vi "Catapult Control Single Solenoid.vi"(6 "Sensor Analog Status":sgl=5.0 format="%#_13g", 7 "Sensor Digital Status":bool, 8 "Error In":errorcluster, 9 "Second Action":T1=enum."Hold", 10 "First Action":T1=enum."Hold", 11 "CatapultDevRefIn":T2={"Catapult State Reference"=refnum, "SolenoidDevRef"={"DevStatus"={"status"=FALSE, "code"=0, "source"=""}, "Pneumatics Control Module"=208, "Forward Solenoid Channel"=enum."Invalid", "Reverse Solenoid Channel"=enum."Invalid"}, "Catapult Configuration Reference"=refnum}) -> (1 "Action Complete":bool=TRUE, 2 "Solenoid Position":bool, 3 "CatapultDevRefOut":T2={"Catapult State Reference"=refnum, "SolenoidDevRef"={"DevStatus"={"status"=FALSE, "code"=0, "source"=""}, "Pneumatics Control Module"=208, "Forward Solenoid Channel"=enum."Invalid", "Reverse Solenoid Channel"=enum."Invalid"}, "Catapult Configuration Reference"=refnum})   [LabVIEW 2015]
uses:
  <userlib>/836 Library/Pneumatics/Catapult/836_CatapultActions.ctl
  <userlib>/836 Library/Pneumatics/Catapult/836_CatapultDevRef.ctl
  <userlib>/836 Library/Pneumatics/Catapult/Catapult State.ctl
  <userlib>/836 Library/Pneumatics/Catapult/CatapultStateMachine.ctl
  <vilib>/Rock Robotics/WPI/Solenoid/WPI_SolenoidDevRef.ctl
  <vilib>/Rock Robotics/WPI/Solenoid/WPI_SolenoidChannel.ctl
  <userlib>/836 Library/Pneumatics/Catapult/Catapult Configuration.ctl
  <vilib>/Rock Robotics/WPI/Solenoid/WPI_SolenoidValue.ctl
  <vilib>/Rock Robotics/WPI/Solenoid/WPI_SolenoidSetEnum.vi
panel:
  out "Error Out":errorcluster
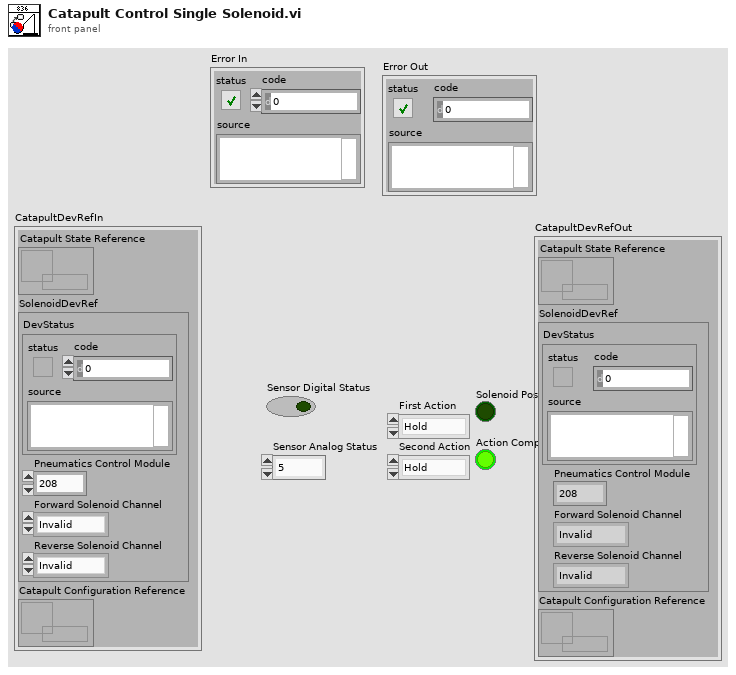
[diagram p1: front panel]
types:
  T1 = typedef "836_CatapultActions.ctl" = enum8{"Fire", "Fire Timed", "Fire Analog", "Fire Digital", "Retract", "Retract Timed", "Retract Analog", "Retract Digital", "Hold", "Toggle", "Toggle Timed", "Toggle Analog", "Toggle Digital"}
  T2 = typedef "836_CatapultDevRef.ctl" = cluster{"Catapult State Reference":refnum<data-value>, "SolenoidDevRef":T3, "Catapult Configuration Reference":refnum<data-value>}
  T3 = typedef "WPI_SolenoidDevRef.ctl" = cluster{"DevStatus":errorcluster, "Pneumatics Control Module":u8, "Forward Solenoid Channel":T4, "Reverse Solenoid Channel":T4}
  T4 = typedef "WPI_SolenoidChannel.ctl" = enum8{"Solenoid 0", "Solenoid 1", "Solenoid 2", "Solenoid 3", "Solenoid 4", "Solenoid 5", "Solenoid 6", "Solenoid 7", "Invalid"}
  T5 = typedef "WPI_SolenoidValue.ctl" = enum16{"Off", "On", "Forward", "Reverse"}
  T6 = typedef "CatapultStateMachine.ctl" = enum8{"Status", "Forward", "Back", "Timed Forward", "Timed Back", "Analog Forwad", "Analog Back", "Digital Forward", "Digital Back", "Off"}
  T7 = typedef "Catapult State.ctl" = cluster{"Position":bool, "Initialize":bool, "First Action?":bool, "Current State":T6, "Multiuse Timer":u32, "Second Action":T1}
  T8 = typedef "Catapult Configuration.ctl" = cluster{"Time Forward":u32, "Time Back":u32, "Digital Forward Samples":u32, "Digital Backward Samples":u32, "Analog Forward Settling Time":u32, "Analog Backward Settling Time":u32, "Analog Forward Threshold":sgl, "Analog Backward Threshold":sgl}
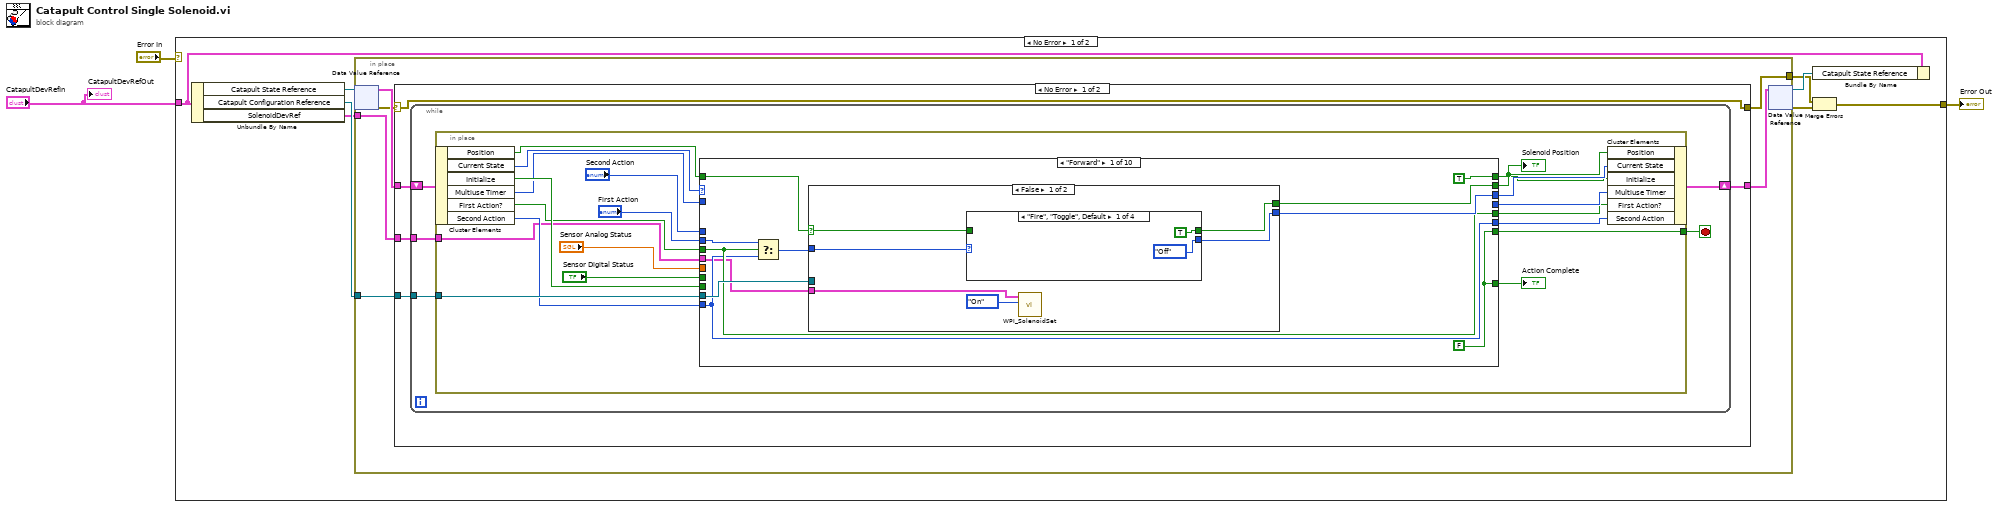
[diagram p0: block diagram]
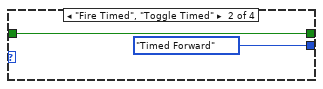
[diagram p2: hidden frame]
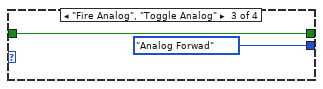
[diagram p3: hidden frame]
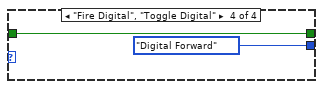
[diagram p4: hidden frame]
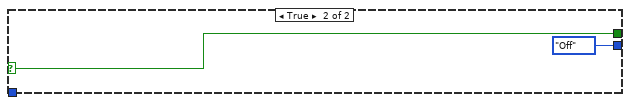
[diagram p5: hidden frame]
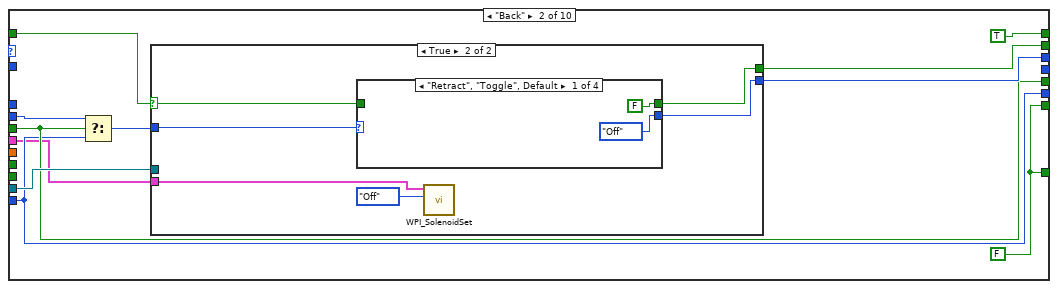
[diagram p6: hidden frame]
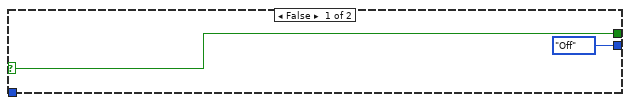
[diagram p7: hidden frame]
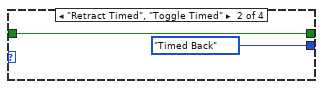
[diagram p8: hidden frame]
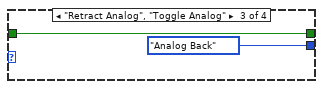
[diagram p9: hidden frame]
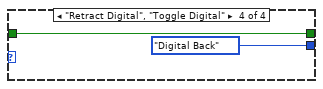
[diagram p10: hidden frame]
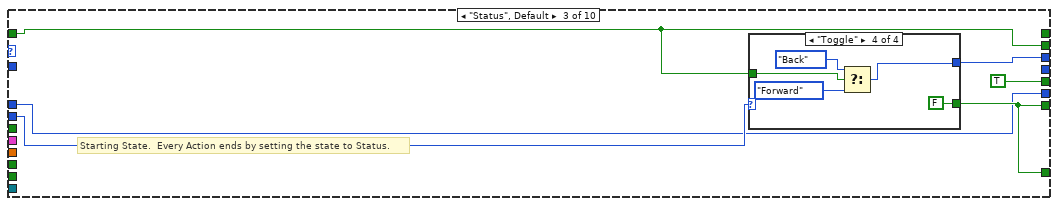
[diagram p11: hidden frame]
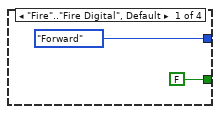
[diagram p12: hidden frame]
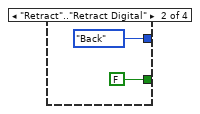
[diagram p13: hidden frame]
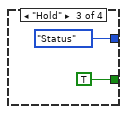
[diagram p14: hidden frame]
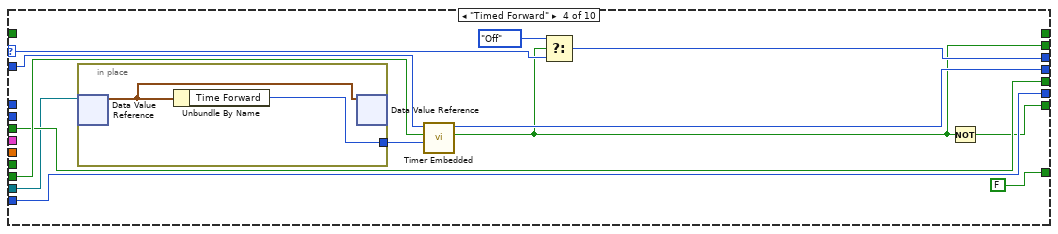
[diagram p15: hidden frame]
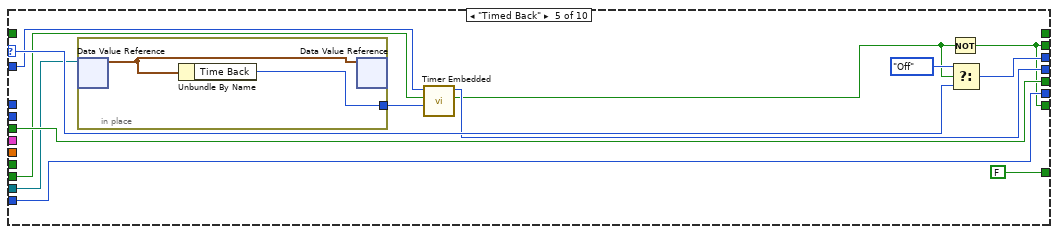
[diagram p16: hidden frame]
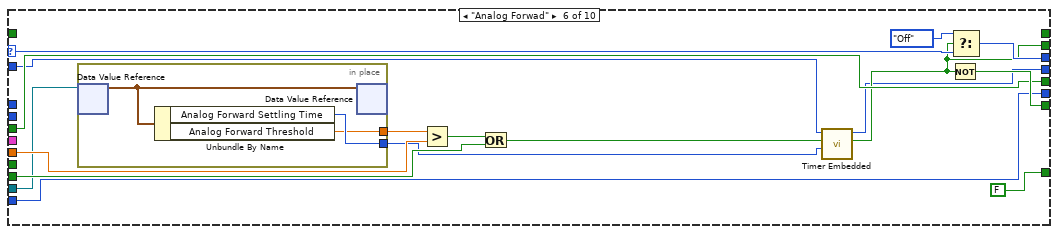
[diagram p17: hidden frame]
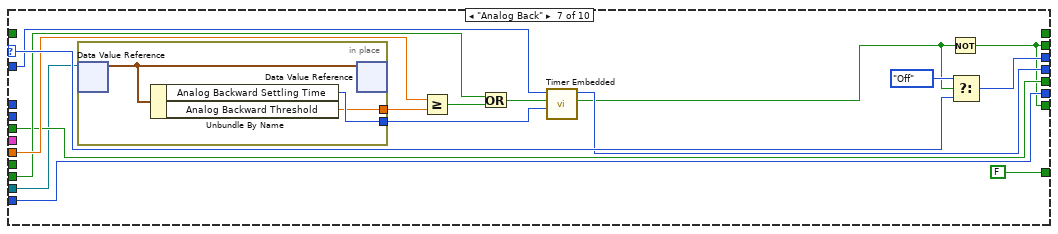
[diagram p18: hidden frame]
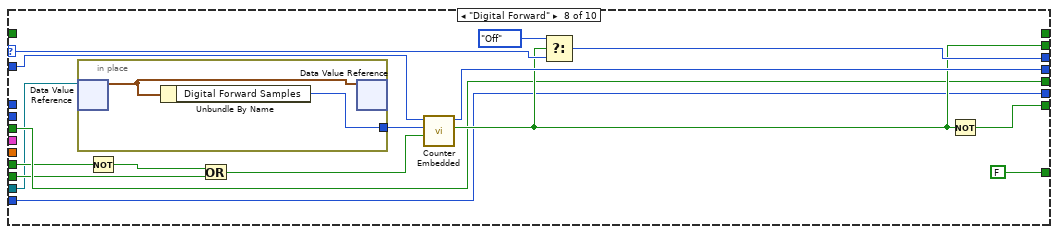
[diagram p19: hidden frame]
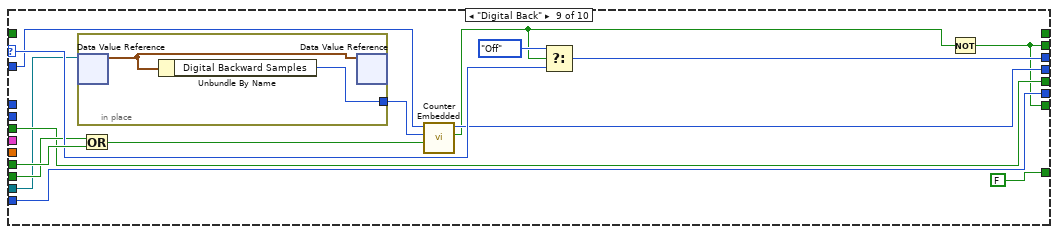
[diagram p20: hidden frame]
diagram:
  n1 = case shown="No Error" "Error In" {
    selector: "Error In" -> [_ w241]
    tunnel: "CatapultDevRefIn" -> [w8 _]
    tunnel: [w5 w241] -> w2
    frame No Error {
      n2 = Unbundle By Name(w8) -> ("Catapult State Reference"=w11:refnum<data-value>, "Catapult Configuration Reference"=w10:refnum<data-value>, "SolenoidDevRef"=w4:T3)
      n3 = in-place {
        in-place-border: w10 -> [w16]
        in-place-border: [w13] -> w7
        in-place-border: w4 -> [w12]
        n4 = in-place-dvr #1(w11) -> (w17:T7, w14:errorcluster)
        n5 = case shown="No Error" w14 {
          selector: w14 -> [w20 w239]
          tunnel: w17 -> [w22 w240]
          tunnel: w16 -> [w21 _]
          tunnel: [w19 w240] -> w15
          tunnel: [w20 w239] -> w13
          tunnel: w12 -> [w18 _]
          frame No Error {
            n6 = while {
              tunnel: w21 -> [w26]
              shift-right: [w24] -> w19
              shift-left: w22 -> [w27]
              tunnel: w18 -> [w23]
              stop <- w25 stop-if-true
              n7 = in-place {
                in-place-border: w26 -> [w40]
                in-place-border: [w36] -> w25
                in-place-border: w23 -> [w28]
                n8 = in-place-cluster #2(w27) -> ("Position"=w44:bool, "Current State"=w38:T6, "Initialize"=w43:bool, "Multiuse Timer"=w39:u32, "First Action?"=w31:bool, "Second Action"=w34:T1)
                n9 = case shown="\"Forward\"" w38 {
                  selector: w38 -> [_ _ _ w130 w145 w162 w184 w202 w218 _]
                  tunnel: [w49 w76 w105 w122 w136 w159 w172 w197 w209 w230] -> w36
                  tunnel: w44 -> [w56 w84 w102 _ _ _ _ _ _ w232]
                  tunnel: [w58 w85 w102 w121 w136 w153 w172 w198 w209 w232] -> w42
                  tunnel: "Sensor Digital Status" -> [_ _ _ _ _ _ _ w193 w220 _]
                  tunnel: [w57 w83 w106 w131 w146 w165 w185 w204 w221 w231] -> w41
                  tunnel: "Sensor Analog Status" -> [_ _ _ _ _ w164 w183 _ _ _]
                  tunnel: w43 -> [_ _ _ w126 w140 w160 w180 w191 w217 _]
                  tunnel: [w49 w76 w105 FALSE FALSE FALSE FALSE FALSE FALSE w230] -> w45
                  tunnel: w39 -> [_ _ _ w127 w139 w155 w175 w199 w213 _]
                  tunnel: [_ _ _ w128 w138 w152 w174 w200 w211 _] -> w35
                  tunnel: w40 -> [w55 w82 _ w120 w135 w151 w171 w190 w208 _]
                  tunnel: [TRUE TRUE _ _ _ _ _ _ _ TRUE] -> w37
                  tunnel: "First Action" -> [w53 w80 w107 _ _ _ _ _ _ _]
                  tunnel: w34 -> [w50 w77 _ w123 w141 w156 w177 w194 w214 w226]
                  tunnel: [w51 w78 TRUE w124 w142 w157 w178 w195 w215 FALSE ("First Action?")] -> w32
                  tunnel: w31 -> [w51 w78 _ w124 w142 w157 w178 w195 w215 w224]
                  tunnel: "Second Action" -> [_ _ w103 _ _ _ _ _ _ _]
                  tunnel: [w50 w77 w103 w123 w141 w156 w177 w194 w214 w226] -> w29
                  tunnel: w28 -> [w48 w75 _ _ _ _ _ _ _ _]
                  frame "Forward" {
                    w49 = FALSE
                    n10 = Select(t=w53, s=w51, f=w50) -> (s? t:f=w52:T1)
                    n11 = case shown="False" w56 {
                      selector: w56 -> [w62 w74]
                      tunnel: [w64 w74] -> w58
                      tunnel: [w63 CatapultStateMachine."Off" ("f")] -> w57
                      tunnel: w55 -> [_ _]
                      tunnel: w52 -> [w60 _]
                      tunnel: w48 -> [w59 _]
                      frame False {
                        n12 = case shown="\"Fire\", \"Toggle\", Default" w60 {
                          tunnel: [CatapultStateMachine."Off" ("Current State") CatapultStateMachine."Timed Forward" ("Current State") CatapultStateMachine."Analog Forwad" ("Current State") CatapultStateMachine."Digital Forward" ("Current State")] -> w63
                          tunnel: w62 -> [_ w68 w70 w72]
                          tunnel: [TRUE w68 w70 w72] -> w64
                          frame "Fire", "Toggle", Default {
                          }
                          frame "Fire Timed", "Toggle Timed" {
                          }
                          frame "Fire Analog", "Toggle Analog" {
                          }
                          frame "Fire Digital", "Toggle Digital" {
                          }
                        }
                        n13 = call-poly <vilib>:"WPI_SolenoidSet.vi"("Value"=WPI_SolenoidValue."On" ("Value 3"), "SolenoidDevRef"=w59) -> ()  [unwired: 8 in, 2 out]
                      }
                      frame True {
                      }
                    }
                  }
                  frame "Back" {
                    w76 = FALSE
                    n14 = Select(t=w80, s=w78, f=w77) -> (s? t:f=w79:T1)
                    n15 = case shown="True" w84 {
                      selector: w84 -> [w87 w91]
                      tunnel: [w87 w93] -> w85
                      tunnel: [CatapultStateMachine."Off" ("f") w92] -> w83
                      tunnel: w82 -> [_ _]
                      tunnel: w79 -> [_ w89]
                      tunnel: w75 -> [_ w88]
                      frame False {
                      }
                      frame True {
                        n16 = case shown="\"Retract\", \"Toggle\", Default" w89 {
                          tunnel: [CatapultStateMachine."Off" ("Current State") CatapultStateMachine."Timed Back" ("Current State") CatapultStateMachine."Analog Back" ("Current State") CatapultStateMachine."Digital Back" ("Current State")] -> w92
                          tunnel: [FALSE w97 w99 w101] -> w93
                          tunnel: w91 -> [_ w97 w99 w101]
                          frame "Retract", "Toggle", Default {
                          }
                          frame "Retract Timed", "Toggle Timed" {
                          }
                          frame "Retract Analog", "Toggle Analog" {
                          }
                          frame "Retract Digital", "Toggle Digital" {
                          }
                        }
                        n17 = call-poly <vilib>:"WPI_SolenoidSet.vi"("Value"=WPI_SolenoidValue."Off" ("Value 3"), "SolenoidDevRef"=w88) -> ()  [unwired: 8 in, 2 out]
                      }
                    }
                  }
                  frame "Status", Default {
                    # "Starting State.  Every Action ends by setting the state to Status."
                    n18 = case shown="\"Toggle\"" w107 {
                      tunnel: [CatapultStateMachine."Forward" ("Current State") CatapultStateMachine."Back" ("Current State") CatapultStateMachine."Status" ("Current State") w114] -> w106
                      tunnel: [FALSE FALSE TRUE FALSE] -> w105
                      tunnel: w102 -> [_ _ _ w117]
                      frame "Fire".."Fire Digital", Default {
                      }
                      frame "Retract".."Retract Digital" {
                      }
                      frame "Hold" {
                      }
                      frame "Toggle" {
                        n19 = Select(t=CatapultStateMachine."Back" ("Current State"), s=w117, f=CatapultStateMachine."Forward" ("Current State")) -> (s? t:f=w114:T6)
                      }
                    }
                  }
                  frame "Timed Forward" {
                    n20 = in-place {
                      in-place-border: [w133] -> w119
                      n21 = in-place-dvr #3(w120) -> (w132:T8)  [unwired: 1 out]
                      n22 = Unbundle By Name(w132) -> ("Time Forward"=w133:u32)
                      n23 = in-place-dvr #3(w132) -> ()  [unwired: 2 out]
                    }
                    n24 = call <userlib>:"Timer Embedded.vi"("Time Limit"=w119, "Reset"=w126, "Start Time In"=w127) -> ("Time Limit Passed"=w121:bool, "Start Time Out"=w128:u32)  [unwired: 7 in]
                    n25 = Select(t=CatapultStateMachine."Off" ("Current State"), s=w121, f=w130) -> (s? t:f=w131:T6)
                    n26 = Not(x=w121) -> (.not. x?=w122:bool)
                  }
                  frame "Timed Back" {
                    n27 = in-place {
                      in-place-border: [w148] -> w134
                      n28 = in-place-dvr #4(w135) -> (w147:T8)  [unwired: 1 out]
                      n29 = Unbundle By Name(w147) -> ("Time Back"=w148:u32)
                      n30 = in-place-dvr #4(w147) -> ()  [unwired: 2 out]
                    }
                    n31 = call <userlib>:"Timer Embedded.vi"("Time Limit"=w134, "Reset"=w140, "Start Time In"=w139) -> ("Time Limit Passed"=w137:bool, "Start Time Out"=w138:u32)  [unwired: 7 in]
                    n32 = Not(x=w137) -> (.not. x?=w136:bool)
                    n33 = Select(t=CatapultStateMachine."Off" ("Current State"), s=w137, f=w145) -> (s? t:f=w146:T6)
                  }
                  frame "Analog Forwad" {
                    n34 = in-place {
                      in-place-border: [w168] -> w150
                      in-place-border: [w167] -> w149
                      n35 = in-place-dvr #5(w151) -> (w166:T8)  [unwired: 1 out]
                      n36 = Unbundle By Name(w166) -> ("Analog Forward Settling Time"=w168:u32, "Analog Forward Threshold"=w167:sgl)
                      n37 = in-place-dvr #5(w166) -> ()  [unwired: 2 out]
                    }
                    n38 = Greater?(x=w149, y=w164) -> (0:w163:bool)
                    n39 = Or(x=w163, y=w160) -> (x .or. y?=w154:bool)
                    n40 = call <userlib>:"Timer Embedded.vi"("Time Limit"=w150, "Reset"=w154, "Start Time In"=w155) -> ("Time Limit Passed"=w153:bool, "Start Time Out"=w152:u32)  [unwired: 7 in]
                    n41 = Not(x=w153) -> (.not. x?=w159:bool)
                    n42 = Select(t=CatapultStateMachine."Off" ("Current State"), s=w153, f=w162) -> (s? t:f=w165:T6)
                  }
                  frame "Analog Back" {
                    n43 = in-place {
                      in-place-border: [w188] -> w169
                      in-place-border: [w187] -> w170
                      n44 = in-place-dvr #6(w171) -> (w186:T8)  [unwired: 1 out]
                      n45 = Unbundle By Name(w186) -> ("Analog Backward Settling Time"=w188:u32, "Analog Backward Threshold"=w187:sgl)
                      n46 = in-place-dvr #6(w186) -> ()  [unwired: 2 out]
                    }
                    n47 = Greater Or Equal?(x=w183, y=w170) -> (x >= y?=w182:bool)
                    n48 = Or(x=w180, y=w182) -> (x .or. y?=w176:bool)
                    n49 = call <userlib>:"Timer Embedded.vi"("Time Limit"=w169, "Reset"=w176, "Start Time In"=w175) -> ("Time Limit Passed"=w173:bool, "Start Time Out"=w174:u32)  [unwired: 7 in]
                    n50 = Not(x=w173) -> (.not. x?=w172:bool)
                    n51 = Select(t=CatapultStateMachine."Off" ("Current State"), s=w173, f=w184) -> (s? t:f=w185:T6)
                  }
                  frame "Digital Forward" {
                    n52 = in-place {
                      in-place-border: [w206] -> w189
                      n53 = in-place-dvr #7(w190) -> (w205:T8)  [unwired: 1 out]
                      n54 = Unbundle By Name(w205) -> ("Digital Forward Samples"=w206:u32)
                      n55 = in-place-dvr #7(w205) -> ()  [unwired: 2 out]
                    }
                    n56 = Not(x=w193) -> (.not. x?=w192:bool)
                    n57 = Or(x=w192, y=w191) -> (x .or. y?=w203:bool)
                    n58 = call <userlib>:"Counter Embedded.vi"("Reset"=w203, "Digital Limit"=w189, "Digital Count In"=w199) -> ("Limit Reached"=w198:bool, "Digital Count Out"=w200:u32)  [unwired: 7 in]
                    n59 = Select(t=CatapultStateMachine."Off" ("Current State"), s=w198, f=w202) -> (s? t:f=w204:T6)
                    n60 = Not(x=w198) -> (.not. x?=w197:bool)
                  }
                  frame "Digital Back" {
                    n61 = in-place {
                      in-place-border: [w223] -> w207
                      n62 = in-place-dvr #8(w208) -> (w222:T8)  [unwired: 1 out]
                      n63 = Unbundle By Name(w222) -> ("Digital Backward Samples"=w223:u32)
                      n64 = in-place-dvr #8(w222) -> ()  [unwired: 2 out]
                    }
                    n65 = Or(x=w217, y=w220) -> (x .or. y?=w212:bool)
                    n66 = call <userlib>:"Counter Embedded.vi"("Reset"=w212, "Digital Limit"=w207, "Digital Count In"=w213) -> ("Limit Reached"=w210:bool, "Digital Count Out"=w211:u32)  [unwired: 7 in]
                    n67 = Select(t=CatapultStateMachine."Off" ("Current State"), s=w210, f=w218) -> (s? t:f=w221:T6)
                    n68 = Not(x=w210) -> (.not. x?=w209:bool)
                  }
                  frame "Off" {
                    n69 = Select(t=w226, s=w224, f=836_CatapultActions."Hold") -> (s? t:f=w227:T1)
                    n70 = case shown="\"Hold\"" w227 {
                      tunnel: [CatapultStateMachine."Forward" ("Current State") CatapultStateMachine."Back" ("Current State") CatapultStateMachine."Status" ("Current State")] -> w231
                      tunnel: [FALSE FALSE TRUE] -> w230
                      frame "Fire".."Fire Digital", Default {
                      }
                      frame "Retract".."Retract Digital" {
                      }
                      frame "Hold" {
                      }
                    }
                  }
                }
                "Solenoid Position" <- w42
                "Action Complete" <- w45
                n71 = in-place-cluster #2("Position"=w42, "Current State"=w41, "Initialize"=w37, "Multiuse Timer"=w35, "First Action?"=w32, "Second Action"=w29) -> (w24:T7)
              }
            }
          }
          frame Error {
          }
        }
        n72 = in-place-dvr #1(w15) -> (w9:refnum<data-value>, w6:errorcluster)
      }
      n73 = Bundle By Name(cluster=w8, "Catapult State Reference"=w9) -> ()  [unwired: 1 out]
      n74 = Merge Errors(w7, w6) -> (w5:errorcluster)
    }
    frame Error {
    }
  }
  "Error Out" <- w2
  "CatapultDevRefOut" <- "CatapultDevRefIn"
